vi "Number to Match.vi"() -> ()   [LabVIEW 2025]
panel:
  in  "?":bool
  out "Iteration Count":i32
  in  "Number to Match":dbl
  # "ME 235: Design of Microprocessor Based Mechanical Systems"
  # "Lab 1 - Number to Match"
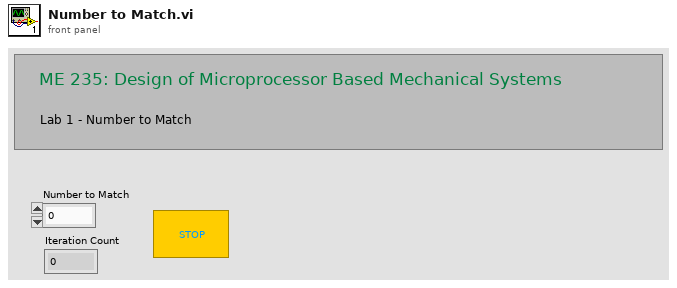
[diagram p1: front panel]
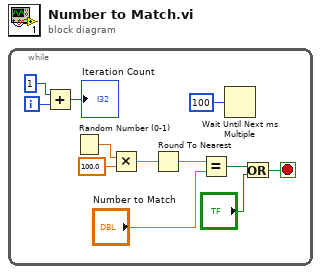
[diagram p0: block diagram]
diagram:
  n1 = while {
    i -> [w11]
    stop <- w2 stop-if-true
    n2 = Add(x=1, y=w11) -> (x+y=→"Iteration Count":i32)
    n3 = Random Number (0-1)() -> (number: 0 to 1=w4:dbl)
    n4 = Multiply(x=w4, y=100.0) -> (x*y=w5:dbl)
    n5 = Round To Nearest(number=w5) -> (nearest integer value=w6:dbl)
    n6 = Equal?(x=w6, y="Number to Match") -> (x = y?=w8:bool)
    n7 = Wait Until Next ms Multiple(millisecond multiple=u32 100) -> ()  [unwired: 1 out]
    n8 = Or(x=w8, y="?") -> (x .or. y?=w2:bool)
  }
